vi "Interleave 2 channel data.vi"(9 "Input Valid":bool=TRUE, 11 "Raw Data":i16[](array[numeric])=[0, 0, 0, 0, 0, 0, 0, 0]) -> (1 "Output Valid":bool=TRUE, 3 "Interleaved Data":i16[](array[numeric]))   [LabVIEW 2012]
doc: "This VI interleaves data from 2 channels. Each channel has 4 samples in parallel."
uses:
  <vilib>/rvi/FXPMathLib/basic elements/FxpDiscreteDelay/XNode/nifxpmath_DiscreteDelay.xnode
panel:
  # "This VI interleaves data from 2 channels. Each channel has 4 samples in parallel."
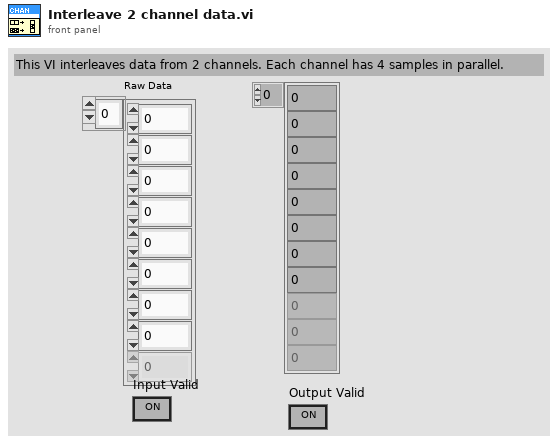
[diagram p1: front panel]
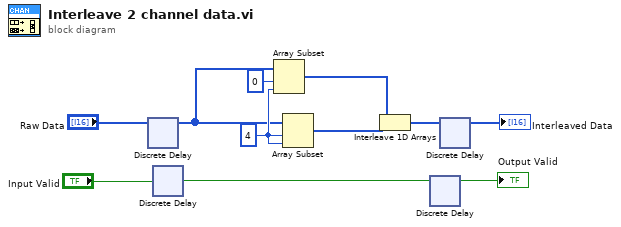
[diagram p0: block diagram]
diagram:
  w10 = 4 ("index")
  n1 = xnode "Discrete Delay"("D"="Raw Data") -> ("Q"=w4:i16[])
  n2 = xnode "Discrete Delay"("D"="Input Valid") -> ("Q"=w2:bool)
  n3 = Array Subset(array=w4, index=0, length=w10) -> (w6:i16[])
  n4 = Array Subset(array=w4, index=w10, length=w10) -> (w9:i16[])
  n5 = Interleave 1D Arrays(w6, w9) -> (w7:i16[])
  n6 = xnode "Discrete Delay"("D"=w2) -> ("Q"=→"Output Valid":bool)
  n7 = xnode "Discrete Delay"("D"=w7) -> ("Q"=→"Interleaved Data":i16[])
